vi "two.vi"   [LabVIEW 2024]
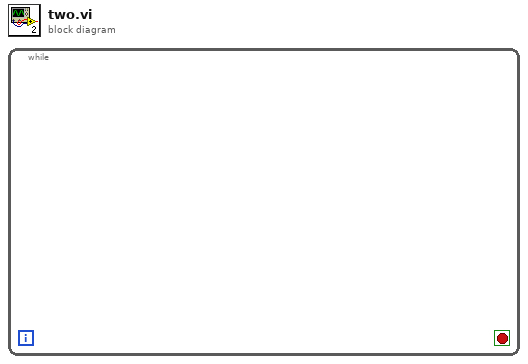
[diagram p0: block diagram]
diagram:
  n1 = while {
    stop <- _ stop-if-true
  }
